vi "Velocity Trapizoid.vi"(8 "Period":i32, 9 "Distance":dbl, 10 "Velocity Max":dbl, 11 "Acceleration Max":dbl) -> (2 "Velocity values":dbl[](array[numeric]), 3 "Timestamp":dbl[](array[numeric]) format="%.2f")   [LabVIEW 2023]
panel:
  out "Time":sgl
  out "XY Graph":cluster{dbl[], dbl[]}(graph)
  out "Time(othy) (in seconds)":dbl
  # "*timeothy is the point where the slope changes in a trapezoid"
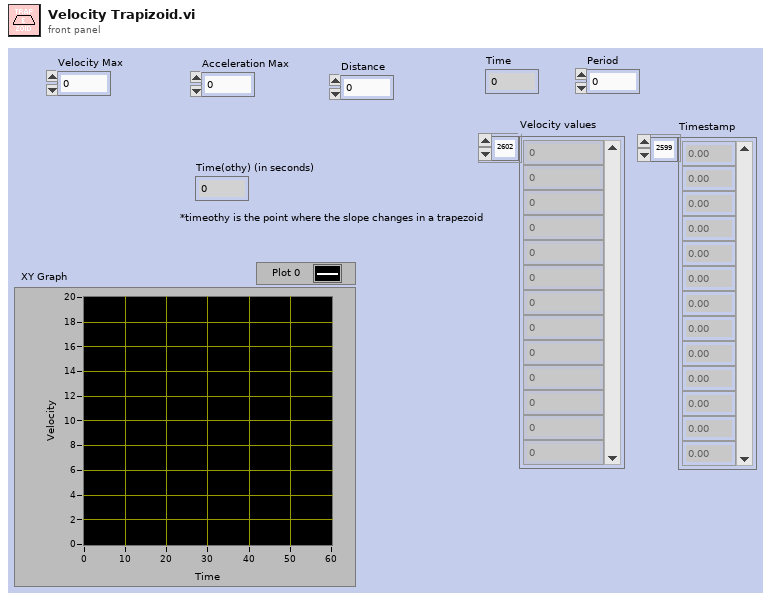
[diagram p1: front panel]
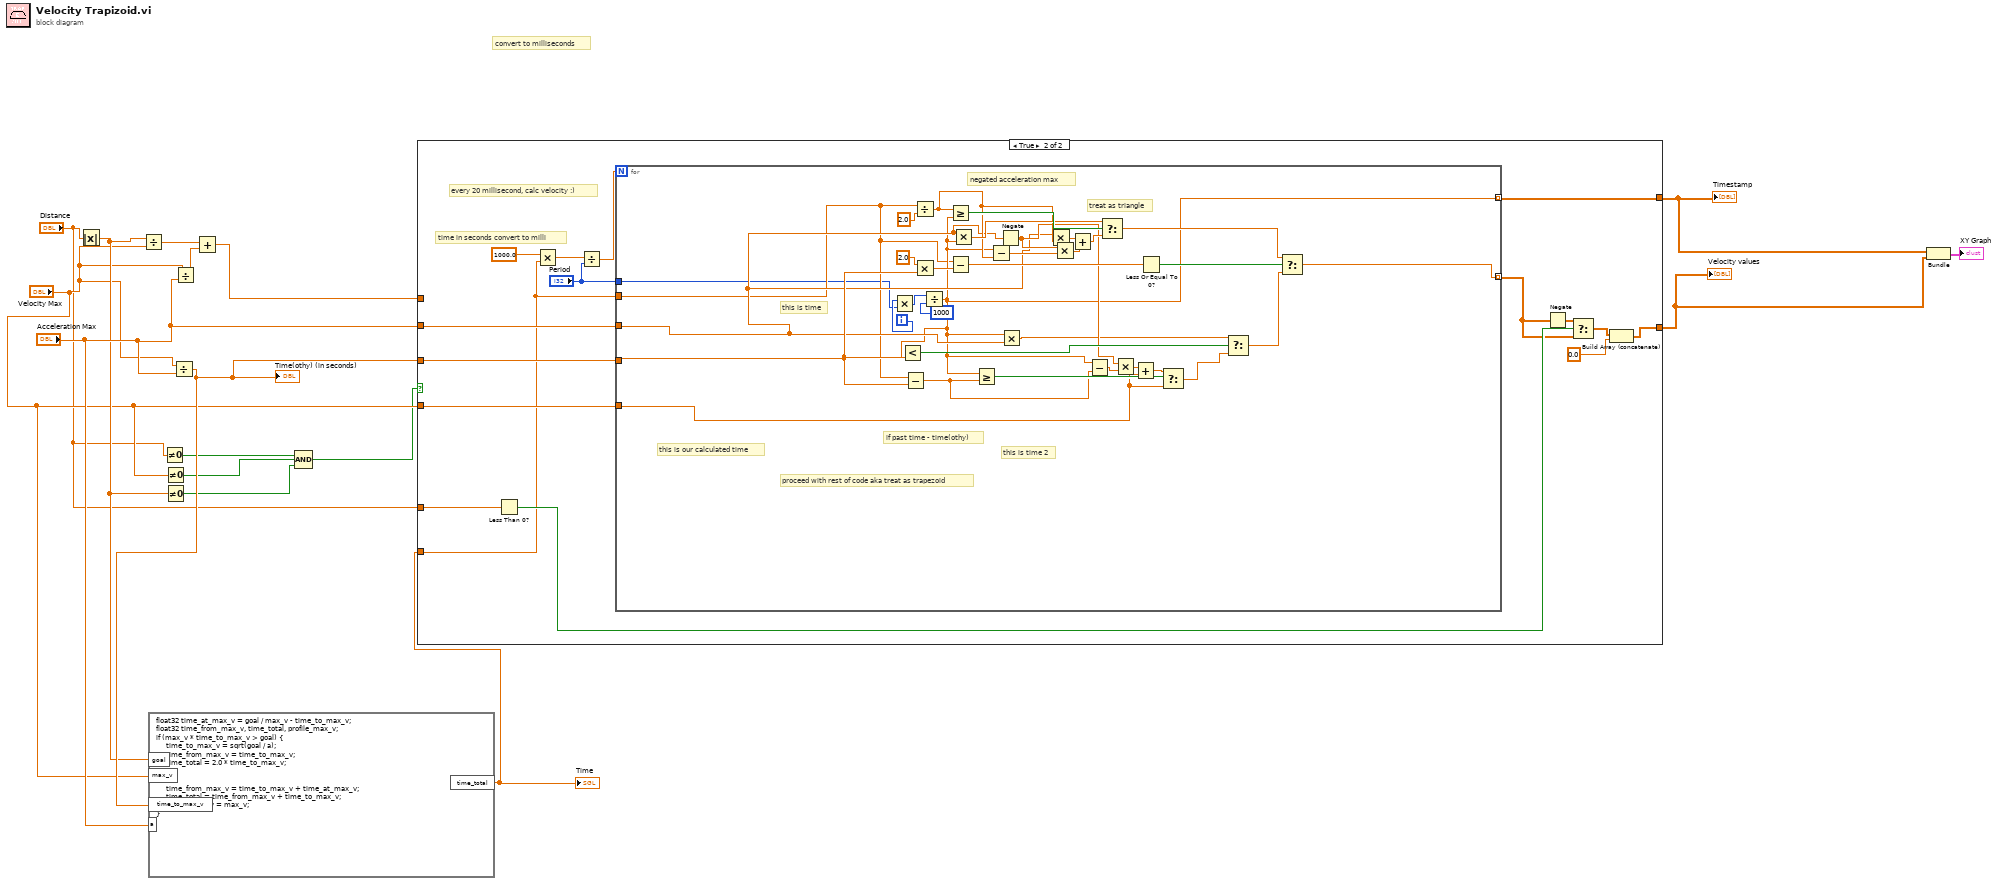
[diagram p0: block diagram]
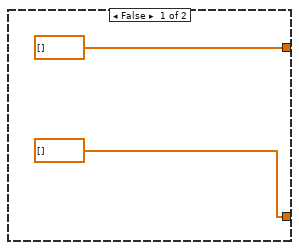
[diagram p2: hidden frame]
diagram:
  # "convert to milliseconds"
  n1 = Absolute Value(x="Distance") -> (abs(x)=w7:dbl)
  n2 = Divide(x=w7, y="Velocity Max") -> (x/y=w13:dbl)
  n3 = Not Equal To 0?(x="Distance") -> (x != 0?=w3:bool)
  n4 = Not Equal To 0?(x="Velocity Max") -> (x != 0?=w2:bool)
  n5 = Not Equal To 0?(x=w7) -> (x != 0?=w1:bool)
  n6 = Divide(x="Velocity Max", y="Acceleration Max") -> (x/y=w8:dbl)
  "Time(othy) (in seconds)" <- w8
  n7 = formula code="float32 time_at_max_v = goal / max_v - time_to_max_v;\nfloat32 time_from_max_v, time_total, profile_max_v;\nif (max_v * time_to_max_v > goal) {\n     time_to_max_v = sqrt(goal / a);\n     time_from_max_v = time_to_max_v;\n     time_total = 2.0 * time_to_max_v;\n}\nelse {\n     time_from_max_v = time_to_max_v + time_at_max_v;\n     time_total = time_from_max_v + time_to_max_v;\n     profile_max_v = max_v;\n}"("goal"=w7, "max_v"="Velocity Max", "time_to_max_v"=w8, "a"="Acceleration Max") -> ("time_total"=w10:sgl)
  "Time" <- w10
  n8 = Divide(x="Velocity Max", y="Acceleration Max") -> (x/y=w16:dbl)
  n9 = Add(x=w13, y=w16) -> (x+y=w14:dbl)
  n10 = Compound Arithmetic op=AND(w3, w2, w1) -> (w4:bool)
  n11 = case shown="True" w4 {
    tunnel: "Velocity Max" -> [_ w34]
    tunnel: w8 -> [_ w33]
    tunnel: [dbl[] [] w20] -> w15
    tunnel: w14 -> [_ _]
    tunnel: "Acceleration Max" -> [_ w31]
    tunnel: [dbl[] [] w21] -> w12
    tunnel: w10 -> [_ w26]
    tunnel: "Distance" -> [_ w27]
    frame False {
    }
    frame True {
      # "every 20 millisecond, calc velocity :)"
      # "time in seconds convert to milli"
      n12 = Less Than 0?(x=w27) -> (x < 0?=w29:bool)
      n13 = Multiply(x=1000.0, y=w26) -> (x*y=w32:dbl)
      n14 = Divide(x=w32, y="Period") -> (x/y=w24:dbl)
      n15 = for {
        N: w24 -> [_]
        tunnel: [w57] -> w28 mode=indexing
        tunnel: w31 -> [w47]
        tunnel: w34 -> [w39]
        tunnel: w33 -> [w56]
        tunnel: [w37] -> w20 mode=indexing
        tunnel: w26 -> [w36]
        tunnel: "Period" -> [w35]
        i -> [w38]
        # "this is our calculated time"
        # "this is time 2"
        # "this is time"
        # "negated acceleration max"
        # "if past time - time(othy)"
        # "treat as triangle"
        # "proceed with rest of code aka treat as trapezoid"
        n16 = Multiply(x=w38, y=w35) -> (x*y=w44:i32)
        n17 = Subtract(x=w36, y=w56) -> (x-y=w45:dbl)
        n18 = Divide(x=w36, y=2.0) -> (x/y=w50:dbl)
        n19 = Multiply(x=2.0, y=w56) -> (x*y=w66:dbl)
        n20 = Divide(x=w44, y=1000) -> (x/y=w37:dbl)
        n21 = Less?(x=w37, y=w56) -> (x < y?=w58:bool)
        n22 = Greater Or Equal?(x=w50, y=w37) -> (x >= y?=w62:bool)
        n23 = Subtract(x=w36, y=w66) -> (x-y=w65:dbl)
        n24 = Multiply(x=w47, y=w37) -> (x*y=w55:dbl)
        n25 = Greater Or Equal?(x=w37, y=w45) -> (x >= y?=w61:bool)
        n26 = Subtract(x=w37, y=w50) -> (x-y=w54:dbl)
        n27 = Negate(x=w47) -> (-x=w49:dbl)
        n28 = Multiply(x=w37, y=w47) -> (x*y=w42:dbl)
        n29 = Multiply(x=w47, y=w50) -> (x*y=w52:dbl)
        n30 = Multiply(x=w49, y=w54) -> (x*y=w53:dbl)
        n31 = Add(x=w52, y=w53) -> (x+y=w51:dbl)
        n32 = Subtract(x=w37, y=w45) -> (x-y=w40:dbl)
        n33 = Select(t=w55, s=w62, f=w51) -> (s? t:f=w46:dbl)
        n34 = Multiply(x=w49, y=w40) -> (x*y=w48:dbl)
        n35 = Add(x=w48, y=w39) -> (x+y=w41:dbl)
        n36 = Less Or Equal To 0?(x=w65) -> (x <= 0?=w64:bool)
        n37 = Select(t=w41, s=w61, f=w39) -> (s? t:f=w60:dbl)
        n38 = Select(t=w42, s=w58, f=w60) -> (s? t:f=w59:dbl)
        n39 = Select(t=w46, s=w64, f=w59) -> (s? t:f=w57:dbl)
      }
      n40 = Negate(x=w28) -> (-x=w30:dbl[])
      n41 = Select(t=w30, s=w29, f=w28) -> (s? t:f=w23:dbl[])
      n42 = Build Array (concatenate)(w23, 0.0) -> (w21:dbl[])
    }
  }
  "Velocity values" <- w12
  "Timestamp" <- w15
  n43 = Bundle(w15, w12) -> (→"XY Graph":cluster{dbl[], dbl[]})  [unwired: 1 in]
